vi "heartBeatWriteCreate.vi"(8 "error in (no error)":errorcluster, 10 "interface object in":refnum<k20>, 11 "MotorController in":refnum<class "MotorController.lvclass">) -> (0 "error out":errorcluster, 2 "interface object out":refnum<k20>, 3 "MotorController out":refnum<class "MotorController.lvclass">)   [LabVIEW 2017]
uses:
  <vilib>/CANopenLib/CANOPEN.llb/CANopen CAN Frame Read Start.vi
  MotorController.lvclass
  <vilib>/CANopenLib/CANOPEN.llb/CANopen CAN Frame Read Create.vi
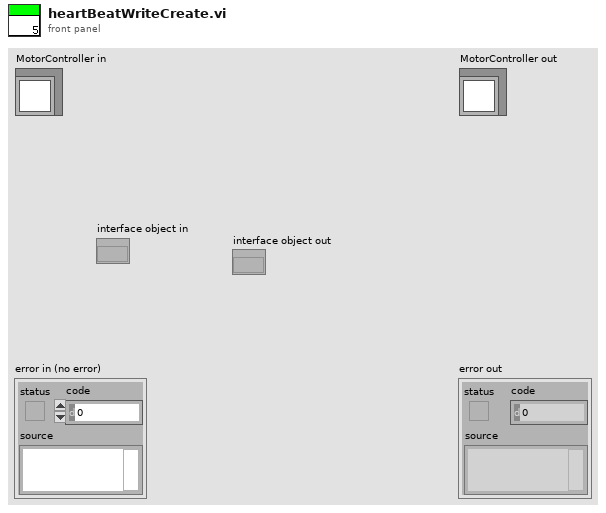
[diagram p1: front panel]
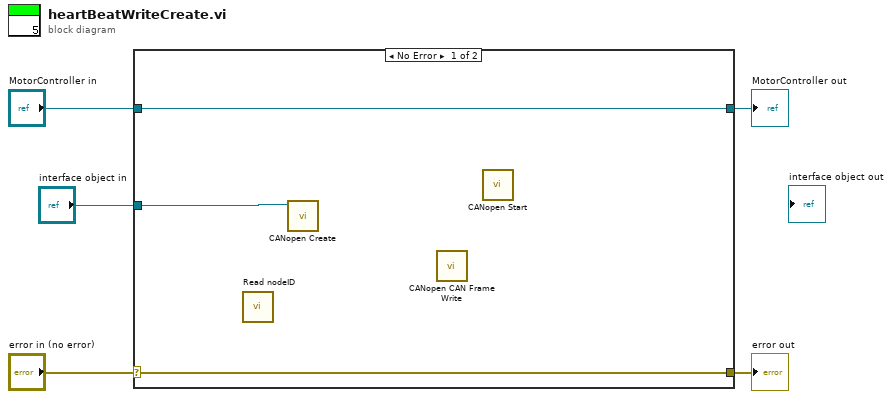
[diagram p0: block diagram]
diagram:
  n1 = case shown="No Error" "error in (no error)" {
    selector: "error in (no error)" -> [w7 w10]
    tunnel: [w7 w10] -> w4
    tunnel: [w8 w9] -> w2
    tunnel: "MotorController in" -> [w8 w9]
    tunnel: "interface object in" -> [w6 _]
    frame No Error {
      n2 = call "Read nodeID.vi"() -> ()  [unwired: 9 in, 3 out]
      n3 = call-poly <vilib>:"CANopen Create.vi"("interface object in"=w6) -> ()  [unwired: 8 in, 3 out]
      n4 = call <vilib>:"CANopen CAN Frame Write.vi"() -> ()  [unwired: 10 in, 2 out]
      n5 = call-poly <vilib>:"CANopen Start.vi"() -> ()  [unwired: 10 in, 2 out]
    }
    frame Error {
    }
  }
  "error out" <- w4
  "MotorController out" <- w2
